vi "Data.Read.vi"(8 "error in":errorcluster, 11 "DVR.state":T2) -> (0 "error out":errorcluster, 1 "changed or first call?":bool, 2 "state":T1)   [LabVIEW 2020]
uses:
  fe013bbb-a456-4d5f-b329-8f8d5fb685ce.vi
  _controls/state.ctl
  _controls/data.ref.ctl
  _controls/data.ctl
  _controls/data.vars.ctl
  _controls/flip.ctl
  <vilib>/vision/Image Controls.llb/IMAQ Image.ctl
  camera/camera.lvclass
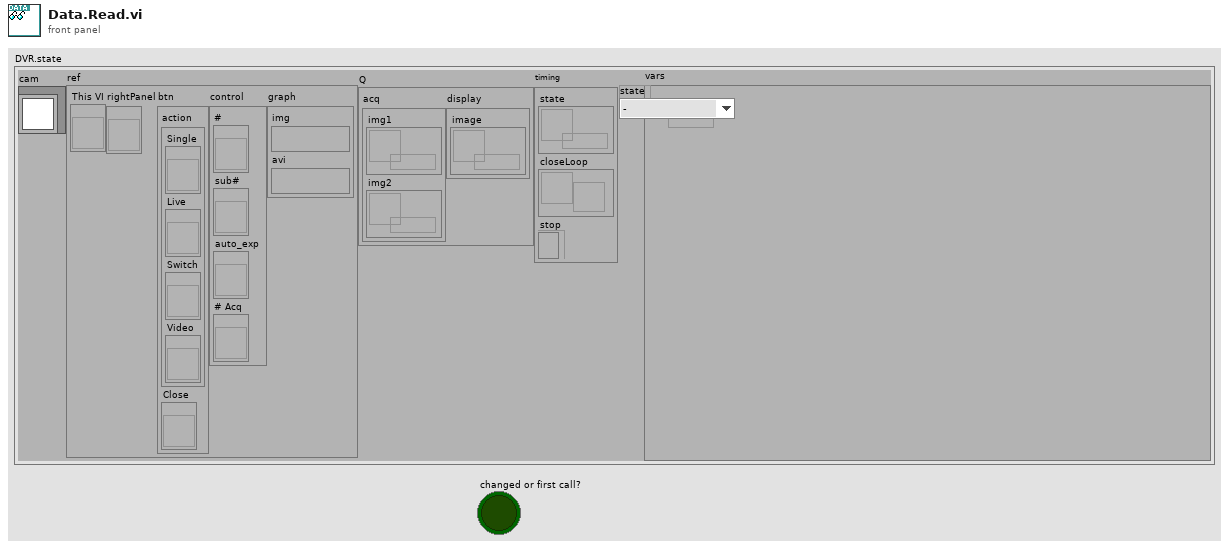
[diagram p1: front panel]
types:
  T1 = typedef "state.ctl" = enum16{"-", "single", "video", "livePL", "PL"}
  T2 = typedef "data.ctl" = cluster{"cam":refnum<class "camera.lvclass">, "ref":T3, "Q":cluster{"acq":cluster{"img1":refnum<queue>, "img2":refnum<queue>}, "display":cluster{"image":refnum<queue>}}, "timing":cluster{"state":refnum<queue>, "closeLoop":refnum<notifier>, "stop":refnum<k4>}, "vars":refnum<data-value>}
  T3 = typedef "data.ref.ctl" = cluster{"This VI":refnum<vi>, "rightPanel":refnum<vi>, "btn":cluster{"action":cluster{"Single":refnum<vi>, "Live":refnum<vi>, "Switch":refnum<vi>, "Video":refnum<vi>}, "Close":refnum<vi>}, "control":cluster{"#":refnum<vi>, "sub#":refnum<vi>, "auto_exp":refnum<vi>, "# Acq":refnum<vi>}, "graph":cluster{"img":T4, "avi":T4}}
  T4 = typedef "IMAQ Image.ctl" = refnum<image>
  T5 = typedef "state.ctl" = enum16{"Init", "default", "single", "LED", "video", "live", "batch", "switching", "update.PL", "update.IR", "stop", "stop2", "quit"}
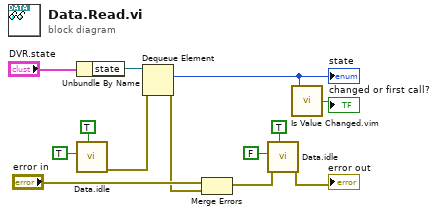
[diagram p0: block diagram]
diagram:
  n1 = Unbundle By Name("DVR.state") -> ("state"=w11:refnum<queue>)
  n2 = call "Data.idle.vi"("write?"=TRUE, "idle in"=TRUE) -> ("error thru"=w7:errorcluster)  [unwired: 8 in, 1 out]
  n3 = Dequeue Element(queue=w11, error in (no error)=w7) -> (element=w1:T5, error out=w10:errorcluster)  [unwired: 1 in, 2 out]
  "state" <- w1
  n4 = Merge Errors("error in", w10) -> (w4:errorcluster)
  n5 = call "Data.idle.vi"("write?"=TRUE, "error in"=w4, "idle in"=FALSE) -> ("error thru"=→"error out":errorcluster)  [unwired: 7 in, 1 out]
  n6 = call "Is Value Changed.vim"("value"=w1) -> ("changed or first call?"=→"changed or first call?":bool)
